vi "Save.vi"(8 "error in":errorcluster, 10 "file path":path, 11 "repository in":refnum<class "NISE_CEF_HierarchyRepo.lvclass">) -> (0 "error out":errorcluster, 3 "repository out":refnum<class "NISE_CEF_HierarchyRepo.lvclass">)   [LabVIEW 2013, in "NISE_CEF_HierarchyRepo.lvclass"]
doc: "Stores repo information to file. It could save in multiple files or formats at the same time. File versioning is suggested."
uses:
  NISE_CEF_HierarchyRepo.lvclass
  Repository/NISE_CEF_Repository.lvclass
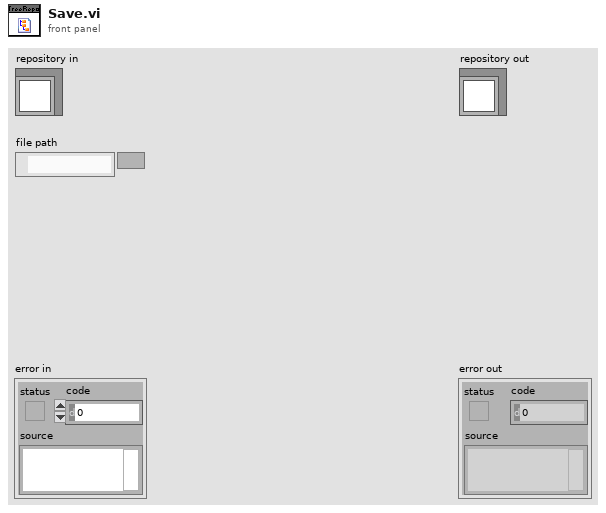
[diagram p1: front panel]
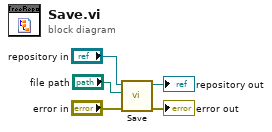
[diagram p0: block diagram]
diagram:
  n1 = call-parent "Save.vi"("error in"="error in", "file path"="file path", "repository in"="repository in") -> ("error out"=→"error out":errorcluster, "repository out"=→"repository out":refnum<class "NISE_CEF_HierarchyRepo.lvclass">)  [unwired: 7 in]
